vi "Get DAQmx Homogeneous Product Name.vi"(11 "Analog source resource names":string[](array[string])) -> (0 "error out":errorcluster, 3 "Device model":string)   [LabVIEW 2021, in "audio adc shared.lvlib"]
uses:
  audio adc shared.lvlib
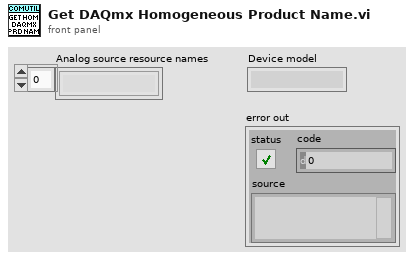
[diagram p1: front panel]
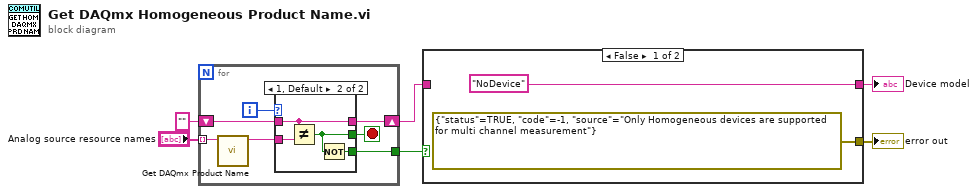
[diagram p0: block diagram]
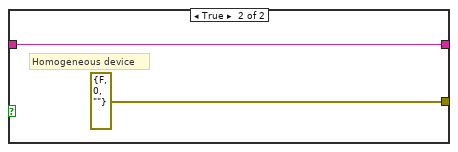
[diagram p2: hidden frame]
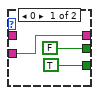
[diagram p3: hidden frame]
diagram:
  n1 = for {
    tunnel: "Analog source resource names" -> [w13] mode=indexing
    shift-right: [w10] -> w2
    shift-left: "" ("DAQmx product type") -> [w9]
    tunnel: [w7] -> w1
    i -> [w12]
    stop <- w8 stop-if-true
    n2 = call "Get DAQmx Product Name.vi"("DAQmx resource name"=w13) -> ("DAQmx product type"=w11:string)  [unwired: 10 in]
    n3 = case shown="1, Default" w12 {
      tunnel: w11 -> [w16 w20]
      tunnel: [w16 w19] -> w10
      tunnel: w9 -> [_ w19]
      tunnel: [FALSE w18] -> w8
      tunnel: [TRUE w17] -> w7
      frame 0 {
      }
      frame 1, Default {
        n4 = Not Equal?(x=w19, y=w20) -> (x != y?=w18:bool)
        n5 = Not(x=w18) -> (.not. x?=w17:bool)
      }
    }
  }
  n6 = case shown="False" w1 {
    tunnel: ["NoDevice" ("f") w23] -> w5
    tunnel: [errorcluster {"status"=TRUE, "code"=-1, "source"="Only Homogeneous devices are supported for multi channel measurement"} ("error constant") errorcluster {"status"=FALSE, "code"=0, "source"=""} ("error constant")] -> w4
    tunnel: w2 -> [_ w23]
    frame False {
    }
    frame True {
      # "Homogeneous device"
    }
  }
  "Device model" <- w5
  "error out" <- w4
